vi "TemperatureSweep.vi"() -> ()   [LabVIEW 2015]
panel:
  out "return count 2":u32
  out "return count":u32
  out "read buffer":string
  out "error out":errorcluster
  in  "error in (no error)":errorcluster
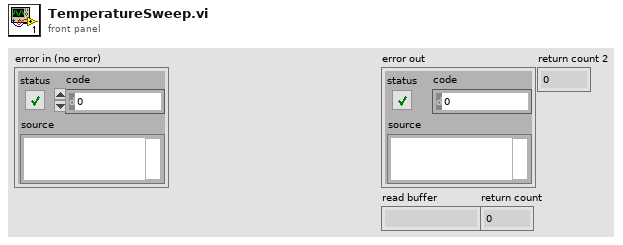
[diagram p1: front panel]
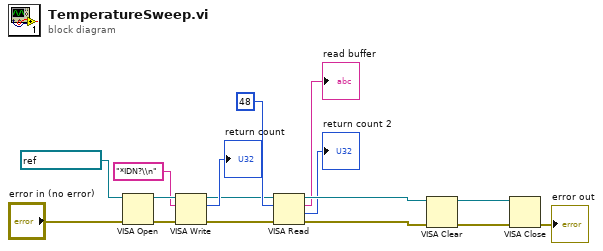
[diagram p0: block diagram]
diagram:
  n1 = VISA Open(error in (no error)="error in (no error)", VISA resource name=refnum<visa-resource-name> "iTC") -> (VISA resource name=w13:refnum<visa-resource-name>, error out=w12:errorcluster)  [unwired: 3 in]
  n2 = VISA Write(VISA resource name=w13, write buffer="*IDN?\\n", error in (no error)=w12) -> (VISA resource name out=w2:refnum<visa-resource-name>, return count=→"return count":u32, error out=w3:errorcluster)
  n3 = VISA Read(VISA resource name=w2, byte count=u32 48, error in (no error)=w3) -> (VISA resource name out=w8:refnum<visa-resource-name>, read buffer=→"read buffer":string, return count=→"return count 2":u32, error out=w7:errorcluster)
  n4 = VISA Clear(VISA resource name=w8) -> (VISA resource name out=w1:refnum<visa-resource-name>)  [unwired: 1 in, 1 out]
  n5 = VISA Close(VISA resource name=w1, error in (no error)=w7) -> (error out=→"error out":errorcluster)
